vi "Method_Const.vi"(4 "Value":u64, 5 "Input A":T1) -> (1 "Result":T1)   [LabVIEW 2021, in "Multiply_U64.lvclass"]
uses:
  Multiply_U64.lvclass
  Abs_Type.ctl
  Abs_Types/U64 Integer/Abs_U64 Integer.lvclass
  C:/TSA/LV_Abstract/Source/Functions/Support/Function/Two Terminal/U64/AbsFunc_Two Term_U64.lvclass
  C:/Program Files (x86)/National Instruments/LabVIEW 2021/vi.lib/TSA/Abstract Data Classes/Abs_Types/U64 Integer/Abs_U64 Integer.lvclass
  Support/Function/Two Terminal/U64/AbsFunc_Two Term_U64.lvclass/AbsFunc_Two Term_U64.ctl
  Support/Function/Two Terminal/U64/Properties/Write Numeric A.vi
  Support/Function/Two Terminal/U64/Properties/Write Numeric B.vi
  Constants/Support/U64/Const_U64.lvclass
  C:/Program Files (x86)/National Instruments/LabVIEW 2021/vi.lib/TSA/Abstract Data Classes/Abs_Types/Numeric/Abs_Numeric.lvclass
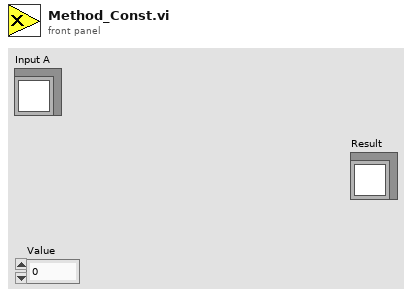
[diagram p1: front panel]
types:
  T1 = typedef "Multiply_U64.lvclass/Abs_Type.ctl" = refnum<class "Abs_U64 Integer.lvclass">
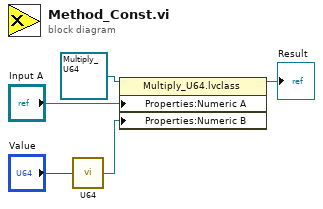
[diagram p0: block diagram]
diagram:
  n1 = call "U64.vi"("Value"="Value") -> ("Constant"=w2:refnum<class "Const_U64.lvclass">)  [unwired: 4 in]
  n2 = property class="Multiply_U64.lvclass"(reference=refnum<class "Multiply_U64.lvclass"> refnum ("Functions.lvlib:Numeric.lvlib:Multiply.lvclass"), "Properties:Numeric A"="Input A", "Properties:Numeric B"=w2) -> (reference out=→"Result":refnum<class "Multiply_U64.lvclass">)  [unwired: 1 in, 1 out]
